vi "Initialize.vi"(8 "error in (no error)":errorcluster, 9 "id query (False)":bool caption="id query (True)", 10 "reset device (False)":bool caption="reset device (True)", 11 "Agilent_3458A in":refnum<class "Agilent_3458.lvclass">) -> (0 "error out":errorcluster, 3 "Agilent_3458A out":refnum<class "Agilent_3458.lvclass">)   [LabVIEW 2018, in "DigitizerPlugins.lvlib" / "Agilent_3458.lvclass"]
uses:
  Agilent_3458.lvclass
  C:/ICDAS/NistPluggableModules/Digitizer/DigitizerPlugins/DigitizerBaseClass/DigitizerBase.lvclass
  DigitizerBaseClass/DigitizerBase.lvclass/DigitizerBase.ctl
  DigitizerBaseClass/Accessors/Read Handle.vi
  DigitizerBaseClass/Accessors/Write InstRef.vi
  <instrlib>/Agilent 3458/Agilent 3458.lvlib
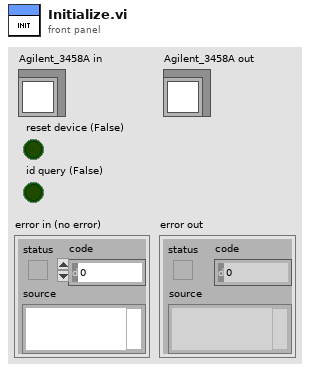
[diagram p1: front panel]
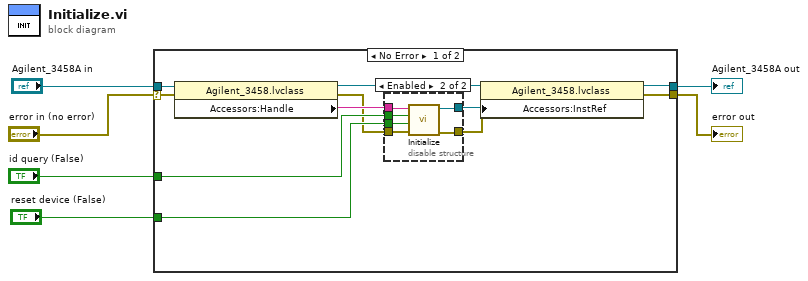
[diagram p0: block diagram]
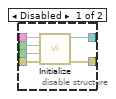
[diagram p2: hidden frame]
diagram:
  n1 = case shown="No Error" "error in (no error)" {
    selector: "error in (no error)" -> [w16 w30]
    tunnel: "Agilent_3458A in" -> [w17 w31]
    tunnel: [w8 w31] -> w4
    tunnel: [w7 w30] -> w3
    tunnel: "id query (False)" -> [w13 _]
    tunnel: "reset device (False)" -> [w12 _]
    frame No Error {
      n2 = property class="Agilent_3458.lvclass"(reference=w17, error in=w16) -> (reference out=w15:refnum<class "Agilent_3458.lvclass">, error out=w11:errorcluster, "Accessors:Handle"=w14:string)
      n3 = disable-structure shown="Enabled" {
        disable-tunnel: w14 -> [w23 w29]
        disable-tunnel: w13 -> [w22 w28]
        disable-tunnel: w12 -> [w21 w27]
        disable-tunnel: w11 -> [w20 w26]
        disable-tunnel: [w19 w24] -> w10
        disable-tunnel: [w18 w25] -> w9
        frame Disabled {
          n4 = call <instrlib>:"Initialize.vi"("error in (no error)"=w20, "Reset (True)"=w21, "ID Query (True)"=w22, "VISA resource name"=w23) -> ("error out"=w18:errorcluster, "VISA resource name out"=w19:refnum<visa-resource-name>)  [unwired: 6 in]
        }
        frame Enabled {
          n5 = call <instrlib>:"Initialize.vi"("error in (no error)"=w26, "Reset (True)"=w27, "ID Query (True)"=w28, "VISA resource name"=w29) -> ("error out"=w25:errorcluster, "VISA resource name out"=w24:refnum<visa-resource-name>)  [unwired: 6 in]
        }
      }
      n6 = property class="Agilent_3458.lvclass"(reference=w15, error in=w9, "Accessors:InstRef"=w10) -> (reference out=w8:refnum<class "Agilent_3458.lvclass">, error out=w7:errorcluster)
    }
    frame Error {
    }
  }
  "error out" <- w3
  "Agilent_3458A out" <- w4
